vi "TDMS Express Write Data (Time and Frequency Domain).vi"() -> ()   [LabVIEW 2023]
doc: "This example demonstrates how to write time-domain and frequency-domain data to a TDMS file using the Write to Measurement File Express VI."
uses:
  Instance           1 61Saved   TDMS - Express write data (time and frequency domain) .vi
  Instance           3 61Saved   TDMS - Express write data (time and frequency domain) .vi
  <vilib>/express/express analysis/Spectral/Block/exnSpectralBlock spectral measurements power poly.vi
  <vilib>/express/express analysis/Spectral/Block/exnSpectralBlock spectral measurements power DDT.vi
  <vilib>/express/express analysis/Spectral/XNode/ExpressSpectralMeasurementsBlockNode.xnode
  <vilib>/Utility/TDMS File Viewer/NI_TDMS File Viewer.lvlib
panel:
  out "Scan number":i32
  out "Power Spectrum":dynamicdata(graph)
  out "Measured Data":dynamicdata(graph)
  # "Overview: Demonstrates how to write time-domain and frequency-domain data to a TDMS file using the Write to Measurement File Express VI.\nInstructions:\n1. Run the VI. It will run for 10 seconds.\n2. When the VI stops, the TDMS file will be displayed in the TDMS File Viewer. In the TDMS File Viewer, right click the graph and select Ignore Time Stamp to view the time waveforms and frequency spectra.\n3. Delete the .tdms file (located at [LabVIEW Data]\\Example Time And Frequency Domain.tdms) when you are done."
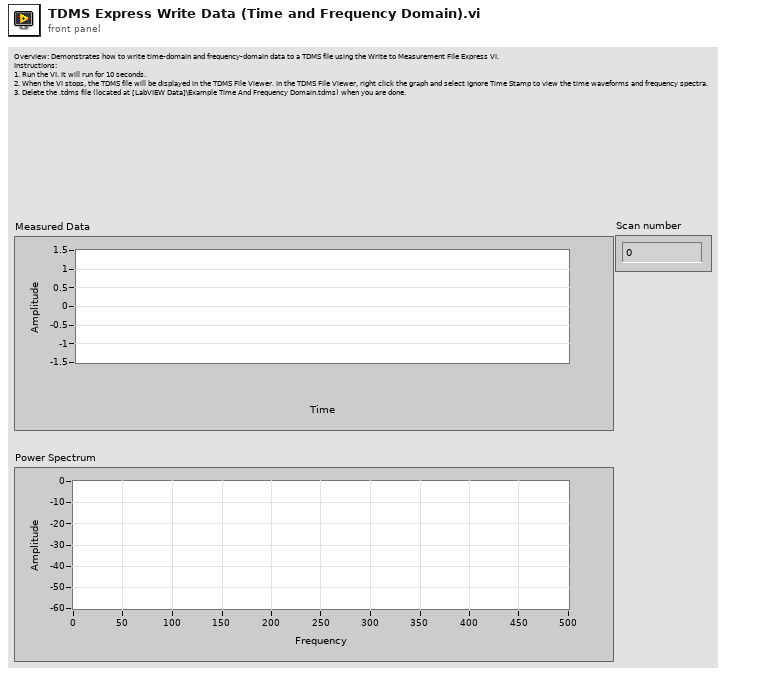
[diagram p1: front panel]
types:
  T1 = cluster{"averaging mode":u16, "weighting mode":u16, "number of averages":u32}
  T2 = cluster{"dB On (F)":bool, "unwrap phase (F)":bool, "convert to degree (F)":bool}
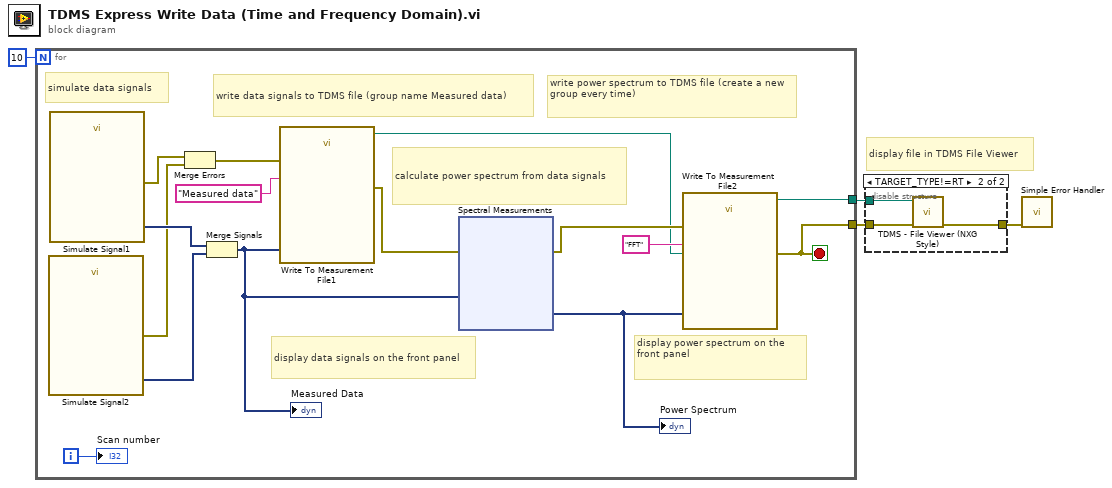
[diagram p0: block diagram]
diagram:
  # "display file in TDMS File Viewer"
  n1 = for {
    N: 10 -> [_]
    tunnel: [w6] -> w4
    tunnel: [w5] -> w2
    i -> [w15]
    stop <- w5 stop-if-true
    # "display power spectrum on the front panel"
    # "display data signals on the front panel"
    # "write power spectrum to TDMS file (create a new group every time)"
    # "calculate power spectrum from data signals"
    # "simulate data signals"
    # "write data signals to TDMS file (group name Measured data)"
    # "Write For Loop"
    n2 = call "Simulate Signal2"() -> ("Square with Uniform Noise"=w18:dynamicdata, "error out"=w11:errorcluster)  [unwired: 9 in, 5 out]
    n3 = call "Simulate Signal1"() -> ("Sine with Uniform Noise"=w19:dynamicdata, "error out"=w12:errorcluster)  [unwired: 8 in, 6 out]
    n4 = Merge Errors(w12, w11) -> (w10:errorcluster)
    n5 = Merge Signals(w19, w18) -> (w17:dynamicdata)
    "Measured Data" <- w17
    n6 = call "Write To Measurement File1"("Signals"=w17, "error in (no error)"=w10, "Comment"="Measured data") -> ("Filename Out"=w7:path, "error out"=w8:errorcluster)  [unwired: 14 in, 1 out]
    n7 = xnode "Spectral Measurements"("Signals"=w17, "error in (no error)"=w8) -> ("Power Spectrum"=w16:dynamicdata, "error out"=w13:errorcluster)
    "Power Spectrum" <- w16
    n8 = call "Write To Measurement File2"("Signals"=w16, "error in (no error)"=w13, "Filename"=w7, "Comment"="FFT") -> ("Filename Out"=w6:path, "error out"=w5:errorcluster)  [unwired: 13 in, 1 out]
    "Scan number" <- w15
  }
  n9 = disable-structure shown="TARGET_TYPE!=RT" {
    disable-tunnel: w4 -> [_ w32]
    disable-tunnel: [w29 w31] -> w3
    disable-tunnel: w2 -> [w29 w30]
    frame condition #0 {
    }
    frame condition #1 (active) {
      n10 = call <vilib>:"TDMS - File Viewer (NXG Style).vi"("error in"=w30, "file in"=w32) -> ("error out"=w31:errorcluster)  [unwired: 8 in, 1 out]
    }
  }
  n11 = call <vilib>:"Simple Error Handler.vi"("error in (no error)"=w3) -> ()  [unwired: 4 in, 5 out]
